vi "start_server.vi"(7 "Running?":refnum<vi>, 8 "error in (no error)":errorcluster, 9 "Max. connection attempts":i32=1000000, 10 "port":u16, 11 "exe directory":path=path "") -> (0 "error out":errorcluster, 3 "connection ID":refnum<k5>)   [LabVIEW 2024]
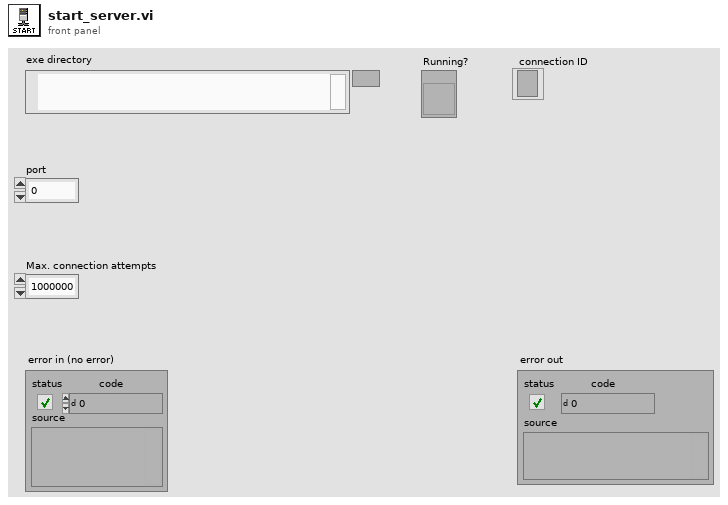
[diagram p1: front panel]
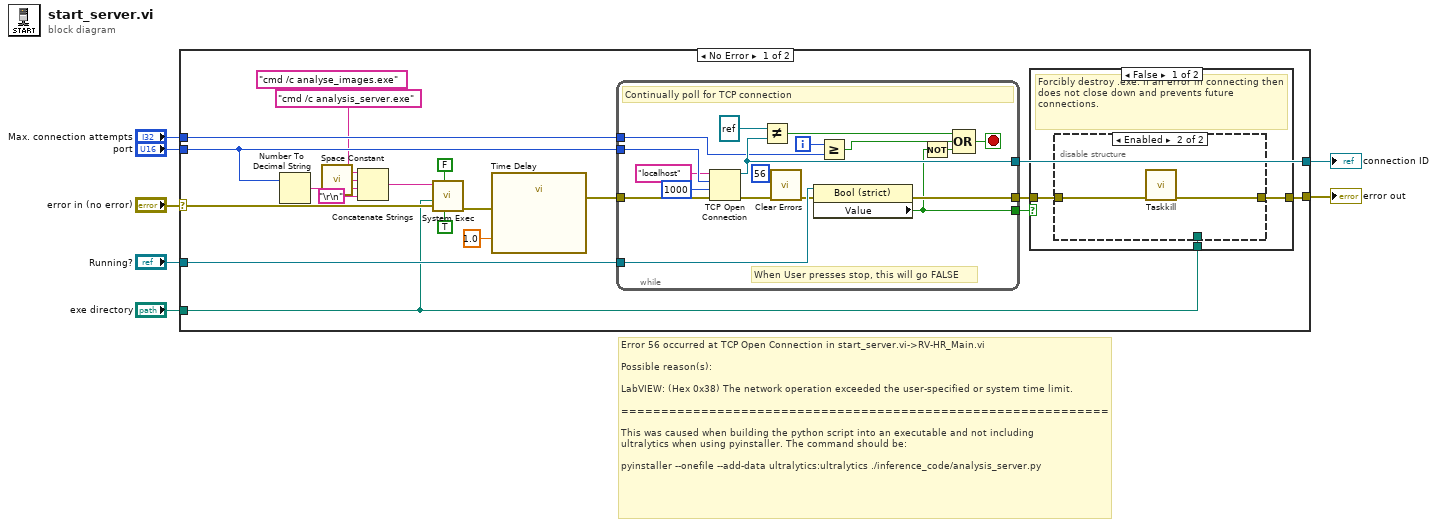
[diagram p0: block diagram]
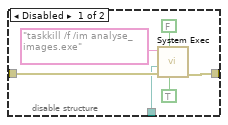
[diagram p2: hidden frame]
diagram:
  # "Error 56 occurred at TCP Open Connection in start_server.vi->RV-HR_Main.vi\n\nPossible reason(s):\n\nLabVIEW: (Hex 0x38) The network operation exceeded the user-specified or system time limit.\n\n=============================================================\n\nThis was caused when building the python script into an executable and not including\nultralytics when using pyinstaller. The command should be:\n\npyinstaller --onefile --add-data ultralytics:ultralytics ./inference_code/analysis_server.py"
  n1 = case shown="No Error" "error in (no error)" {
    selector: "error in (no error)" -> [w26 w57]
    tunnel: [w11 w57] -> w6
    tunnel: "exe directory" -> [w10 _]
    tunnel: "port" -> [w16 _]
    tunnel: "Max. connection attempts" -> [w15 _]
    tunnel: "Running?" -> [w14 _]
    tunnel: [w13 _] -> w1
    frame No Error {
      (unwired) "cmd /c analyse_images.exe" ("string")
      n2 = Number To Decimal String(number=w16) -> (decimal integer string=w22:string)  [unwired: 1 in]
      n3 = call <vilib>:"Space Constant.vi"() -> ("String"=w23:string)
      n4 = Concatenate Strings("cmd /c analysis_server.exe" ("string"), w23, w22, "\r\n") -> (w18:string)
      n5 = call <vilib>:"System Exec.vi"("run minimized? (F)"=TRUE, "wait until completion? (T)"=FALSE, "error in (no error)"=w26, "working directory"=w10, "command line"=w18) -> ("error out"=w20:errorcluster)  [unwired: 3 in, 3 out]
      n6 = call "Time Delay"("error in (no error)"=w20, "Delay Time (s)"=1.0) -> ("error out"=w17:errorcluster)  [unwired: 9 in]
      n7 = while {
        tunnel: w17 -> [w42]
        tunnel: w16 -> [w56]
        tunnel: [w46] -> w12
        tunnel: [w48] -> w13
        tunnel: w15 -> [w47]
        tunnel: w14 -> [w45]
        tunnel: [w44] -> w9
        i -> [w49]
        stop <- w52 stop-if-true
        # "When User presses stop, this will go FALSE"
        # "Continually poll for TCP connection"
        n8 = TCP Open Connection(address="localhost", remote port or service name=w56, timeout ms (60000)=1000, error in (no error)=w42) -> (connection ID=w48:refnum<k5>, error out=w41:errorcluster)  [unwired: 1 in]
        n9 = Not Equal?(x=refnum<k5> refnum ("connection ID"), y=w48) -> (x != y?=w51:bool)
        n10 = call <vilib>:"Clear Errors.vi"("error in (no error)"=w41, "specific error code to clear (0: all)"=56) -> ("error out"=w40:errorcluster)  [unwired: 4 in, 1 out]
        n11 = property class="Bool (strict)"(reference=w45, error in=w40) -> (error out=w46:errorcluster, "Value"=w44:bool)  [unwired: 1 out]
        n12 = Greater Or Equal?(x=w49, y=w47) -> (x >= y?=w50:bool)
        n13 = Not(x=w44) -> (.not. x?=w43:bool)
        n14 = Compound Arithmetic op=OR(w51, w50, w43) -> (w52:bool)
      }
      n15 = case shown="False" w9 {
        tunnel: w12 -> [w29 w38]
        tunnel: [w28 w38] -> w11
        tunnel: w10 -> [w27 _]
        frame False {
          # "Forcibly destroy .exe. If an error in connecting then does not close down and prevents future connections."
          n16 = disable-structure shown="Enabled" {
            disable-tunnel: w29 -> [w32 w37]
            disable-tunnel: [w31 w36] -> w28
            disable-tunnel: w27 -> [w30 _]
            frame Disabled {
              n17 = call <vilib>:"System Exec.vi"("run minimized? (F)"=TRUE, "wait until completion? (T)"=FALSE, "error in (no error)"=w32, "working directory"=w30, "command line"="taskkill /f /im analyse_images.exe") -> ("error out"=w31:errorcluster)  [unwired: 3 in, 3 out]
            }
            frame Enabled {
              n18 = call "Taskkill.vi"("error in (no error)"=w37) -> ("error out"=w36:errorcluster)  [unwired: 9 in, 1 out]
            }
          }
        }
        frame True {
        }
      }
    }
    frame Error {
    }
  }
  "error out" <- w6
  "connection ID" <- w1
